vi "README example set.vi"() -> ()   [LabVIEW 2020]
uses:
  EXT.vi
  String.vi
  2D EXT.vi
  Time Stamp.vi
  1D EXT.vi
  infolib.lvlib
panel:
  out "info data out":string
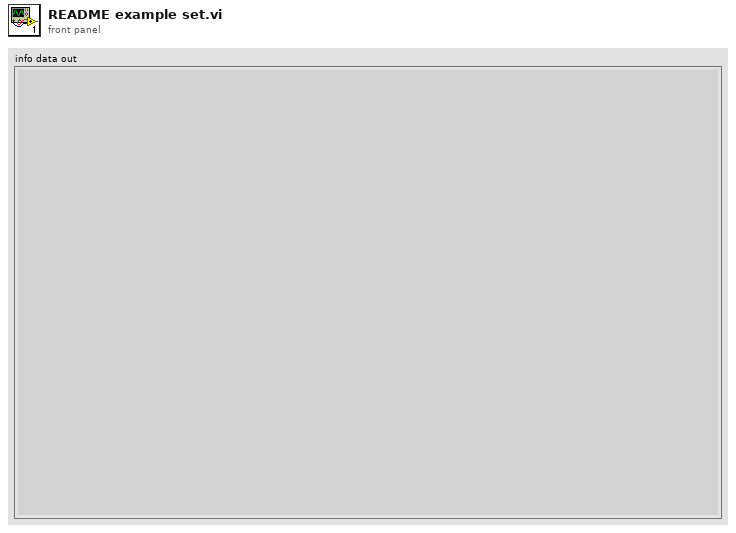
[diagram p1: front panel]
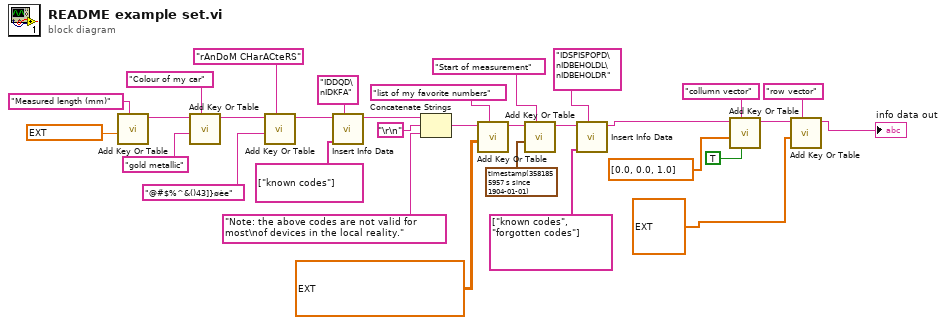
[diagram p0: block diagram]
diagram:
  n1 = call-poly "Add Key Or Table.vi"("key description"="Measured length (mm)", "numeric"=ext 34.123456789) -> ("info data out"=w29:string)  [unwired: 8 in, 1 out]
  n2 = call-poly "Add Key Or Table.vi"("key description"="Colour of my car", "string"="gold metallic" ("key description"), "info data"=w29) -> ("info data out"=w24:string)  [unwired: 7 in, 1 out]
  n3 = call-poly "Add Key Or Table.vi"("key description"="rAnDoM CHarACteRS", "string"="@#$%^&()43]}øèe" ("key description"), "info data"=w24) -> ("info data out"=w23:string)  [unwired: 7 in, 1 out]
  n4 = call "Insert Info Data.vi"("info data to insert"="IDDQD\nIDKFA" ("key description"), "sections"=string[] ["known codes"], "info data"=w23) -> ("info data out"=w20:string)  [unwired: 7 in, 1 out]
  n5 = Concatenate Strings(w20, "\r\n", "Note: the above codes are not valid for most\nof devices in the local reality." ("string")) -> (w17:string)
  n6 = call-poly "Add Key Or Table.vi"("key description"="list of my favorite numbers", "numeric"=ext[][] [[1.0, 11.0, 42.0], [3333.0, 1e+72, 0.0], [-1.0, -3333.0, 0.00000100000000000000000004]], "info data"=w17) -> ("info data out"=w14:string)  [unwired: 7 in, 1 out]
  n7 = call-poly "Add Key Or Table.vi"("key description"="Start of measurement", "time stamp"=timestamp(3581855957.019788 s since 1904-01-01), "info data"=w14) -> ("info data out"=w13:string)  [unwired: 7 in, 1 out]
  n8 = call "Insert Info Data.vi"("info data to insert"="IDSPISPOPD\nIDBEHOLDL\nIDBEHOLDR", "sections"=string[] ["known codes", "forgotten codes"], "info data"=w13) -> ("info data out"=w8:string)  [unwired: 7 in, 1 out]
  n9 = call-poly "Add Key Or Table.vi"("collumn vector (F)"=TRUE, "key description"="collumn vector", "numeric"=dbl[] [0.0, 0.0, 1.0], "info data"=w8) -> ("info data out"=w6:string)  [unwired: 6 in, 1 out]
  n10 = call-poly "Add Key Or Table.vi"("key description"="row vector", "numeric"=ext[] [0.0, 0.0, 1.0], "info data"=w6) -> ("info data out"=→"info data out":string)  [unwired: 7 in, 1 out]
